vi "ResourceVisa1.vi"() -> ()   [LabVIEW 2020]
panel:
  in  "VISA resource name":refnum<visa-resource-name>
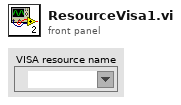
[diagram p1: front panel]
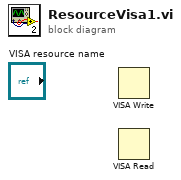
[diagram p0: block diagram]
diagram:
  n1 = VISA Write() -> ()  [unwired: 3 in, 3 out]
  n2 = VISA Read() -> ()  [unwired: 3 in, 4 out]
